vi "Clear DAQmx Tasks.vi"(8 "error in (no error)":errorcluster) -> (0 "error out":errorcluster)   [LabVIEW 2013]
uses:
  Triggers/Globals/gl_Triggering globals.vi
panel:
  out "Array":errorcluster[](array[cluster])
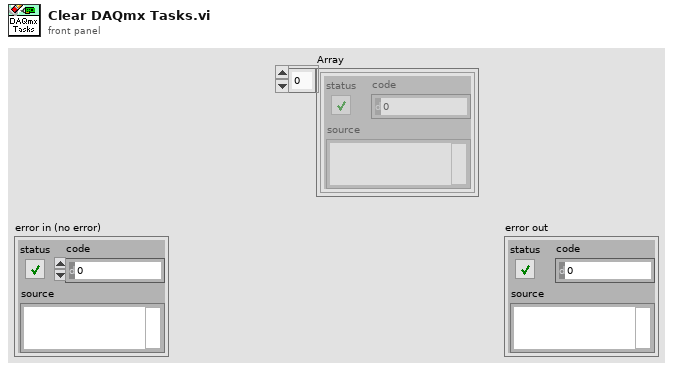
[diagram p1: front panel]
types:
  T1 = typedef "Triggered tasks cluster.ctl" = cluster{"DO task-Encoder trigger":refnum<k21>, "AO Task-Pockels modulation":refnum<k21>, "Counter Clock Task":refnum<k21>}
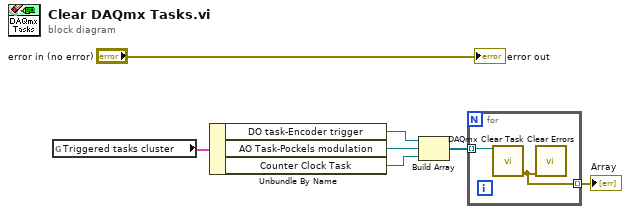
[diagram p0: block diagram]
diagram:
  n1 = global read "gl_Triggering globals.vi" "Triggered tasks cluster"() -> (w6:T1)
  n2 = Unbundle By Name(w6) -> ("DO task-Encoder trigger"=w3:refnum<k21>, "AO Task-Pockels modulation"=w5:refnum<k21>, "Counter Clock Task"=w4:refnum<k21>)
  n3 = Build Array(w3, w5, w4) -> (w2:refnum<k21>[])
  n4 = for {
    tunnel: w2 -> [w9] mode=indexing
    tunnel: [w8] -> w1 mode=indexing
    n5 = call <vilib>:"DAQmx Clear Task.vi"("task in"=w9) -> ("error out"=w8:errorcluster)  [unwired: 14 in]
    n6 = call <vilib>:"Clear Errors.vi"("error in (no error)"=w8) -> ()  [unwired: 6 in, 1 out]
  }
  "Array" <- w1
  "error out" <- "error in (no error)"
